vi "SubVI RX Receiver Close.vi"(0 "硬件设置":T1={"设备IP地址"="192.168.11.3", "选择天线"="RF1", "载波频率(Hz)"=2400000000.0, "增益(dB)"=10.0, "采样时间(s)"=0.0033, "触发电平"=0.01, "带宽(Hz)"=40000000.0, "参考位置(%)"=10.0} {"参考位置(%)" format="%.2p"; "带宽(Hz)" format="%.2p"; "触发电平" format="%.2p"; "采样时间(s)" format="%.2p"; "增益(dB)" format="%.2f"; "载波频率(Hz)" format="%.2p"}, 11 "错误输入":errorcluster) -> (15 "错误输出":errorcluster)   [LabVIEW 2015]
uses:
  SubVI RX HW Parameters.ctl
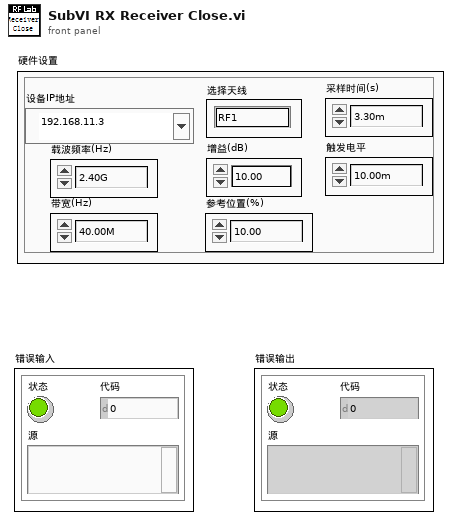
[diagram p1: front panel]
types:
  T1 = typedef "SubVI RX HW Parameters.ctl" = cluster{"设备IP地址":refnum<k15>, "选择天线":string, "载波频率(Hz)":dbl, "增益(dB)":dbl, "采样时间(s)":dbl, "触发电平":dbl, "带宽(Hz)":dbl, "参考位置(%)":dbl}
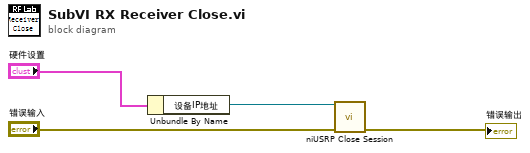
[diagram p0: block diagram]
diagram:
  n1 = Unbundle By Name("硬件设置") -> ("设备IP地址"=w4:refnum<k15>)
  n2 = call <instrlib>:"niUSRP Close Session.vi"("session handle"=w4, "error in (no error)"="错误输入") -> ("error out"=→"错误输出":errorcluster)  [unwired: 13 in]
